vi "Monitor TestStatePTC.vi"(8 "error in (no error)":errorcluster, 10 "Address (0)":i32, 11 "VISA resource name":refnum<visa-resource-name>) -> (0 "error out":errorcluster, 1 "measured humidity":dbl, 2 "measured temp":dbl, 3 "VISA resource name out":refnum<visa-resource-name>, 4 "number of alarms":i32, 5 "Mode":T1, 6 "specimen temp":dbl)   [LabVIEW 2016, in "Environment Chamber.lvlib" / "Climatic Chamber.lvlib"]
doc: "<b>Test area state monitor (incl. specimen Temp.)</B>\n\nReturns the chamber test area state (including specimen temperature control)."
uses:
  Climatic Chamber.lvlib
  Private/Type Defs/Mode Enum.ctl
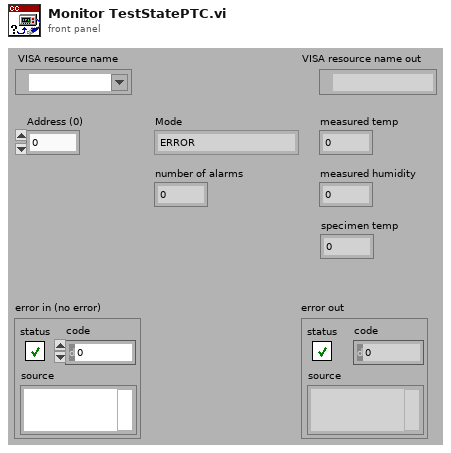
[diagram p1: front panel]
types:
  T1 = typedef "Environment Chamber.lvlib/Climatic Chamber.lvlib/Mode Enum.ctl" = enum16{"ERROR", "OFF", "STANDBY", "CONSTANT", "RUN", "RUN PAUSE", "RUN END HOLD", "RMT RUN", "RMT RUN PAUSE", "RMT RUN END HOLD"}
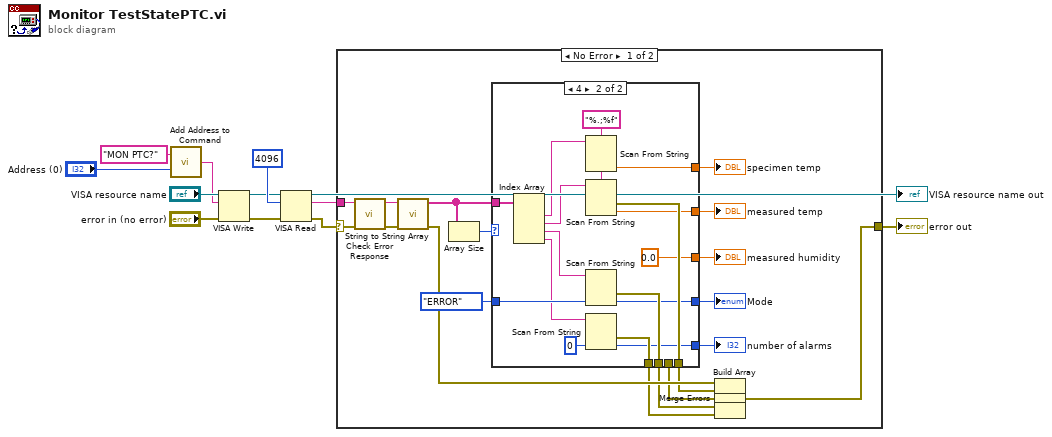
[diagram p0: block diagram]
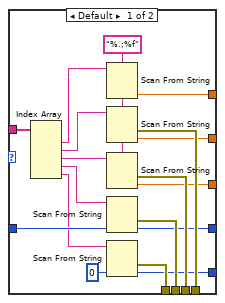
[diagram p2: hidden frame]
diagram:
  n1 = call "Add Address to Command.vi"("Address (0)"="Address (0)", "Command"="MON PTC?") -> ("Command OUT"=w4:string)
  n2 = VISA Write(VISA resource name="VISA resource name", write buffer=w4, error in (no error)="error in (no error)") -> (VISA resource name out=w9:refnum<visa-resource-name>, error out=w8:errorcluster)  [unwired: 1 out]
  n3 = VISA Read(VISA resource name=w9, byte count=u32 4096, error in (no error)=w8) -> (VISA resource name out=→"VISA resource name out":refnum<visa-resource-name>, read buffer=w2:string, error out=w3:errorcluster)  [unwired: 1 out]
  n4 = case shown="No Error" w3 {
    selector: w3 -> [w29 w66]
    tunnel: w2 -> [w31 _]
    tunnel: [w19 w66] -> w1
    frame No Error {
      n5 = call "Check Error Response.vi"("error in (no error)"=w29, "read String"=w31) -> ("error out"=w28:errorcluster, "String out"=w30:string)  [unwired: 7 in, 1 out]
      n6 = call "String to String Array.vi"("error in (no error)"=w28, "String received"=w30) -> ("error out"=w27:errorcluster, "Array Data"=w25:string[])  [unwired: 8 in]
      n7 = Array Size(array=w25) -> (size(s)=w26:i32)
      n8 = case shown="4" w26 {
        tunnel: w25 -> [w45 w62]
        tunnel: [w43 w60] -> w24
        tunnel: [w41 0.0] -> w23
        tunnel: Mode_Enum."ERROR" ("MODE") -> [w39 w59]
        tunnel: [w38 w58] -> w21
        tunnel: [w36 w57] -> w20
        tunnel: [w49 w65] -> w18
        tunnel: [w48 _] -> w17
        tunnel: [w47 w64] -> w16
        tunnel: [w46 w63] -> w15
        tunnel: [w33 w50] -> w14
        frame Default {
          w34 = "%.;%f" ("format string")
          n9 = Index Array(array=w45) -> (element #1=w32:string, element #2=w44:string, element #3=w42:string, element #4=w40:string, element #5=w37:string)  [unwired: 5 in]
          n10 = Scan From String(format string=w34, input string=w32) -> (output 1=w33:dbl)  [unwired: 3 in, 3 out]
          n11 = Scan From String(format string=w34, input string=w44) -> (error out=w49:errorcluster, output 1=w43:dbl)  [unwired: 3 in, 2 out]
          n12 = Scan From String(format string=w34, input string=w42) -> (error out=w48:errorcluster, output 1=w41:dbl)  [unwired: 3 in, 2 out]
          n13 = Scan From String(input string=w40, default 1=w39) -> (error out=w47:errorcluster, output 1=w38:T1)  [unwired: 3 in, 2 out]
          n14 = Scan From String(input string=w37, default 1=0) -> (error out=w46:errorcluster, output 1=w36:i32)  [unwired: 3 in, 2 out]
        }
        frame 4 {
          w51 = "%.;%f" ("format string")
          n15 = Index Array(array=w62) -> (element #1=w52:string, element #2=w61:string, element #3=w55:string, element #4=w54:string)  [unwired: 4 in]
          n16 = Scan From String(format string=w51, input string=w52) -> (output 1=w50:dbl)  [unwired: 3 in, 3 out]
          n17 = Scan From String(format string=w51, input string=w61) -> (error out=w65:errorcluster, output 1=w60:dbl)  [unwired: 3 in, 2 out]
          n18 = Scan From String(input string=w55, default 1=w59) -> (error out=w64:errorcluster, output 1=w58:T1)  [unwired: 3 in, 2 out]
          n19 = Scan From String(input string=w54, default 1=0) -> (error out=w63:errorcluster, output 1=w57:i32)  [unwired: 3 in, 2 out]
        }
      }
      "measured temp" <- w24
      "measured humidity" <- w23
      "Mode" <- w21
      "number of alarms" <- w20
      "specimen temp" <- w14
      n20 = Build Array(w27, w18, w17, w16, w15) -> (w13:errorcluster[])
      n21 = Merge Errors(w13) -> (w19:errorcluster)
    }
    frame Error {
    }
  }
  "error out" <- w1
